vi "Reset Max-Min.vi"(0 "VISA resource name":refnum<visa-resource-name>, 7 "Reset Max/Min (True)":bool=TRUE, 11 "error in (no error)":errorcluster) -> (4 "VISA resource name out":refnum<visa-resource-name>, 15 "error out":errorcluster)   [LabVIEW 2013, in "Lake Shore Cryotronics 331.lvlib"]
doc: "This VI resets Min/Max function for all inputs."
uses:
  Lake Shore Cryotronics 331.lvlib
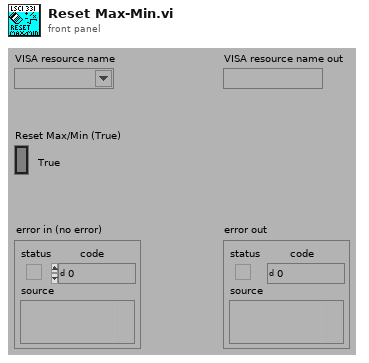
[diagram p1: front panel]
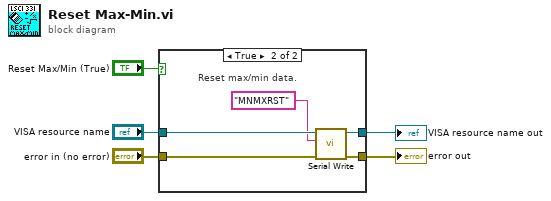
[diagram p0: block diagram]
diagram:
  n1 = case shown="True" "Reset Max/Min (True)" {
    tunnel: "VISA resource name" -> [w7 w12]
    tunnel: "error in (no error)" -> [w6 w11]
    tunnel: [w7 w10] -> w2
    tunnel: [w6 w9] -> w1
    frame False {
      # "Do not reset max/min."
    }
    frame True {
      # "Reset max/min data."
      n2 = call "Serial Write.vi"("error in (no error)"=w11, "Write Buffer (\"\")"="MNMXRST", "VISA resource name"=w12) -> ("error out"=w9:errorcluster, "VISA resource name out"=w10:refnum<visa-resource-name>)  [unwired: 6 in, 1 out]
    }
  }
  "VISA resource name out" <- w2
  "error out" <- w1
